vi "shift register while loop.vi"() -> ()   [LabVIEW 2018]
panel:
  out "Numeric":i32
  out "x+y":i32
  out "Iterations":i32
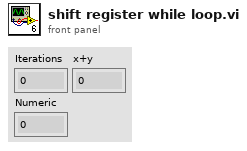
[diagram p1: front panel]
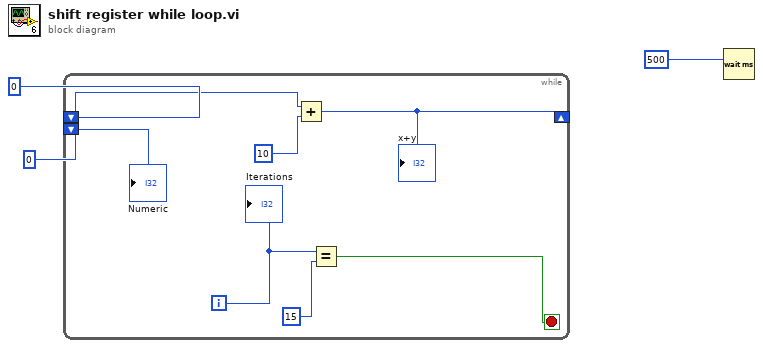
[diagram p0: block diagram]
diagram:
  n1 = while {
    shift-right: [w8] -> _
    shift-left: 0 -> [w9]
    shift-left: 0 -> [w4]
    i -> [w5]
    stop <- w7 stop-if-true
    n2 = Add(x=w9, y=10) -> (x+y=w8:i32)
    "x+y" <- w8
    n3 = Equal?(x=w5, y=15) -> (x = y?=w7:bool)
    "Iterations" <- w5
    "Numeric" <- w4
  }
  n4 = Wait (ms)(milliseconds to wait=500) -> ()  [unwired: 1 out]
